vi "Send alert (SubVI).vi"(0 "Exchange.lvclass":refnum<class "Exchange.lvclass">, 1 "target":string, 2 "Channel in":refnum<class "Channel.lvclass">, 3 "error in (no error)":errorcluster, 4 "alert content":string) -> (6 "error out":errorcluster)   [LabVIEW 2016]
uses:
  <vilib>/Distrio/LabbitMQ/Exchange/Exchange.lvclass
  <vilib>/Distrio/LabbitMQ/Channel/Channel.lvclass
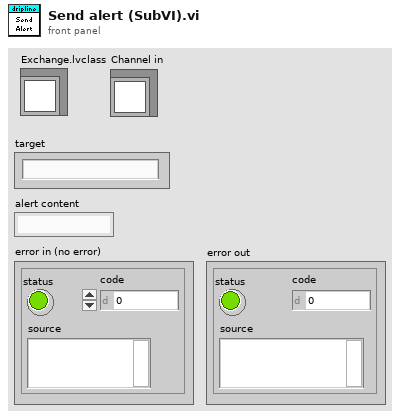
[diagram p1: front panel]
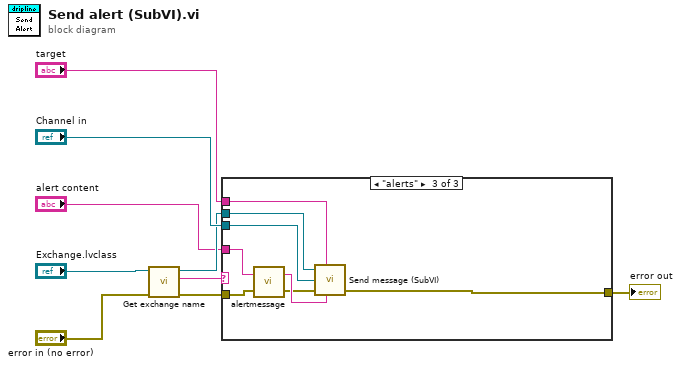
[diagram p0: block diagram]
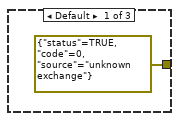
[diagram p2: hidden frame]
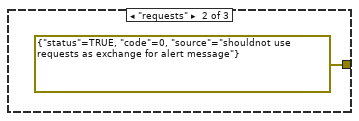
[diagram p3: hidden frame]
diagram:
  n1 = call <vilib>:"Get exchange name.vi"("error in (no error)"="error in (no error)", "Exchange in"="Exchange.lvclass") -> ("error out"=w8:errorcluster, "name"=w4:string, "Exchange out"=w6:refnum<class "Exchange.lvclass">)  [unwired: 7 in]
  n2 = case shown="\"alerts\"" w4 {
    tunnel: "Channel in" -> [_ _ w19]
    tunnel: w8 -> [_ _ w15]
    tunnel: w6 -> [_ _ w18]
    tunnel: "target" -> [_ _ w17]
    tunnel: [errorcluster {"status"=TRUE, "code"=0, "source"="unknown exchange"} ("error constant") errorcluster {"status"=TRUE, "code"=0, "source"="shouldnot use requests as exchange for alert message"} ("error constant") w12] -> w2
    tunnel: "alert content" -> [_ _ w13]
    frame Default {
    }
    frame "requests" {
    }
    frame "alerts" {
      n3 = call "alertmessage.vi"("error in (no error)"=w15, "reply content"=w13) -> ("error out"=w14:errorcluster, "body"=w16:string)
      n4 = call "Send message (SubVI).vi"("Exchange.lvclass"=w18, "target"=w17, "Channel in"=w19, "error in (no error)"=w14, "body"=w16) -> ("error out"=w12:errorcluster)  [unwired: 1 in, 3 out]
    }
  }
  "error out" <- w2
